vi "CHECK QUEUE STATUS.vi"(8 "error in (no error)":errorcluster, 11 "StateAuto in":refnum<class "StateAuto.lvclass">) -> (0 "error out":errorcluster, 2 "stateAuto":T1, 3 "StateAuto out":refnum<class "StateAuto.lvclass">)   [LabVIEW 2017, in "StateAuto.lvclass"]
uses:
  StateAuto.lvclass
  controls/StateMachineAuto.ctl
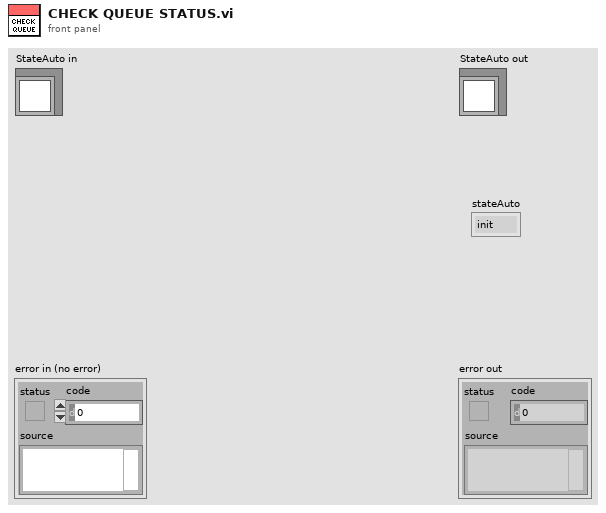
[diagram p1: front panel]
types:
  T1 = typedef "StateMachineAuto.ctl" = enum16{"init", "checkEMG", "checkStateBoard", "checkQueue", "writeDataQueue", "initNextCommand", "endNextCommand"}
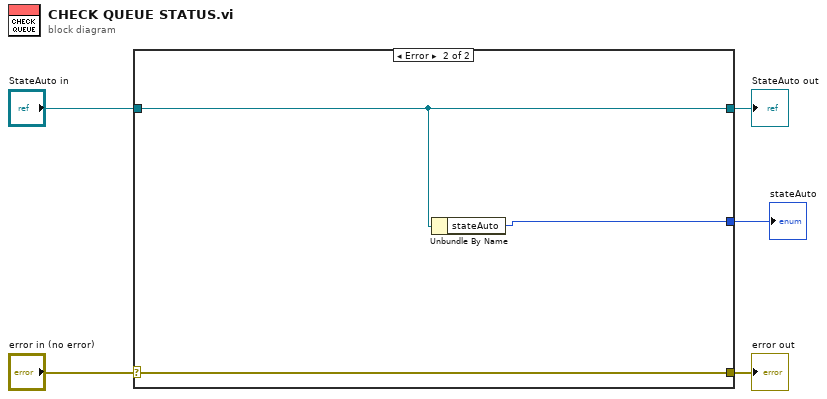
[diagram p0: block diagram]
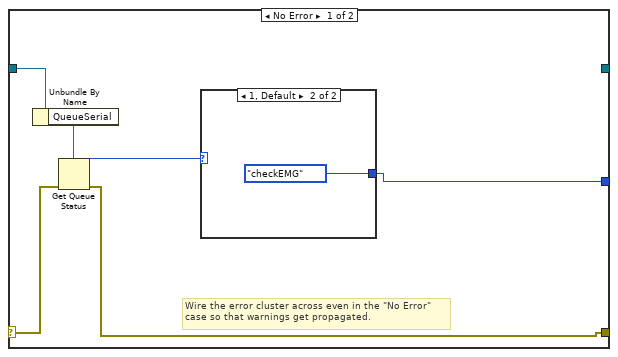
[diagram p2: hidden frame]
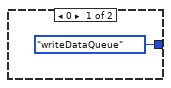
[diagram p3: hidden frame]
diagram:
  n1 = case shown="Error" "error in (no error)" {
    selector: "error in (no error)" -> [w9 w16]
    tunnel: [w8 w16] -> w4
    tunnel: [_ w15] -> w2
    tunnel: "StateAuto in" -> [w7 w15]
    tunnel: [w6 w14] -> w1
    frame No Error {
      # "Wire the error cluster across even in the \"No Error\"\ncase so that warnings get propagated."
      n2 = Unbundle By Name(w7) -> ("QueueSerial"=w11:refnum<queue>)
      n3 = Get Queue Status(queue=w11, error in (no error)=w9) -> (error out=w8:errorcluster, # elements in queue=w10:i32)  [unwired: 1 in, 6 out]
      n4 = case shown="1, Default" w10 {
        tunnel: [StateMachineAuto."writeDataQueue" ("stateAuto") StateMachineAuto."checkEMG" ("stateAuto")] -> w6
        frame 0 {
        }
        frame 1, Default {
        }
      }
    }
    frame Error {
      n5 = Unbundle By Name(w15) -> ("stateAuto"=w14:T1)
    }
  }
  "error out" <- w4
  "StateAuto out" <- w2
  "stateAuto" <- w1
